vi "open-class-private-data-edit-time.vi"(6 "Mouse Position":T1, 7 "User VI Ref":refnum<vi>, 8 "Is Multi-select?":bool, 9 "Remaining Items":refnum<vi>[](array[refnum]), 10 "Affected Items":T8, 11 "Menu Refnum":refnum<k9>) -> (3 "Menu Items To Add":T2[](array[typedef]))   [LabVIEW 2022 SP3]
doc: "This VI is part of a plug-in for modifying the LabVIEW shortcut menus. This is the builder VI which is called when the shortcut menu is built. It tells LabVIEW which shortcut menu items to add to the menu."
uses:
  <resource>/plugins/PopupMenus/support/Checkmark Status.ctl
  <resource>/plugins/PopupMenus/support/Relative Position.ctl
  <resource>/plugins/PopupMenus/support/Position In Menu.ctl
  <resource>/plugins/PopupMenus/support/Transaction Control.ctl
  <resource>/plugins/PopupMenus/support/Shortcut Menu Item Definition.ctl
  <resource>/plugins/PopupMenus/support/Enabled Menu Item Status.ctl
  open-class-private-data-edit-time.ctl
  <vilib>/Utility/miscctls.llb/LVPositionTypeDef.ctl
panel:
  # "Rules a popup plug-in must follow:\n* This VI's file name must match the file name of the LLB -- only the file extensions should be different.\n* This VI must have debugging disabled or it will be ignored as a plug-in.\n* For all menu items, \"tag suffix + file name of this VI\" must be less than 240 characters.\n* You can disconnect the \"Affected Items\" from the typedef to make the plug-in load faster. The typedef is only there to assist you in keeping this VI and the execution VI using to the same type.\n* All controls on this panel except \"Affected Items\" are locked to prevent accidental edits. Do not change the types or the names of controls other than the elements inside the \"Affected Items\" cluster.\n* See Context Help for more information on the individual controls."
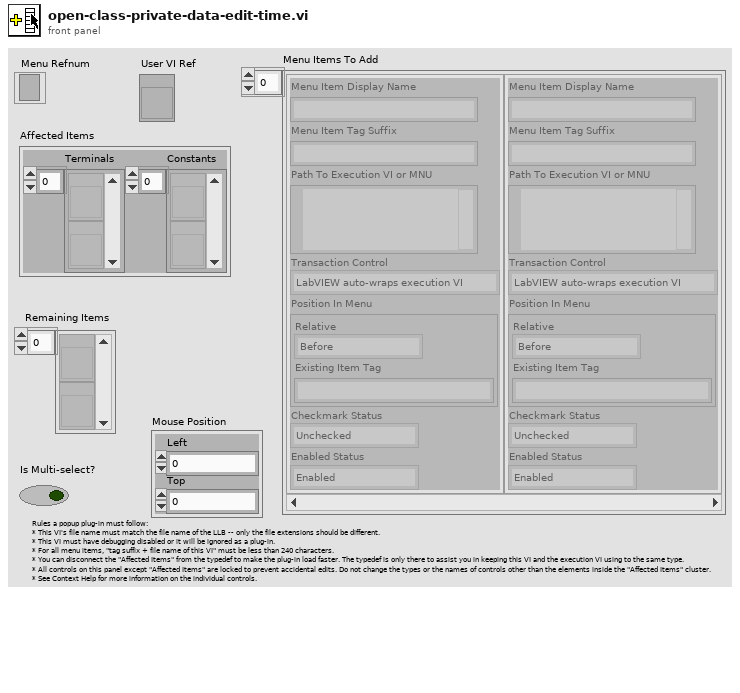
[diagram p1: front panel]
types:
  T1 = typedef "LVPositionTypeDef.ctl" = cluster{"Left":i32, "Top":i32}
  T2 = typedef "Shortcut Menu Item Definition.ctl" = cluster{"Menu Item Display Name":string, "Menu Item Tag Suffix":string, "Path To Execution VI or MNU":path, "Transaction Control":T3, "Position In Menu":T4, "Checkmark Status":T6, "Enabled Status":T7}
  T3 = typedef "Transaction Control.ctl" = enum8{"LabVIEW auto-wraps execution VI", "Execution VI will define if needed"}
  T4 = typedef "Position In Menu.ctl" = cluster{"Relative":T5, "Existing Item Tag":string}
  T5 = typedef "Relative Position.ctl" = enum8{"Before", "Instead of", "After", "Into Submenu"}
  T6 = typedef "Checkmark Status.ctl" = enum8{"Unchecked", "Checked"}
  T7 = typedef "Enabled Menu Item Status.ctl" = enum8{"Enabled", "Disabled"}
  T8 = typedef "open-class-private-data-edit-time.ctl" = cluster{"Terminals":refnum<vi>[], "Constants":refnum<vi>[]}
  T9 = enum32{"not a typedef", "typedef", "strict typedef", "class private data"}
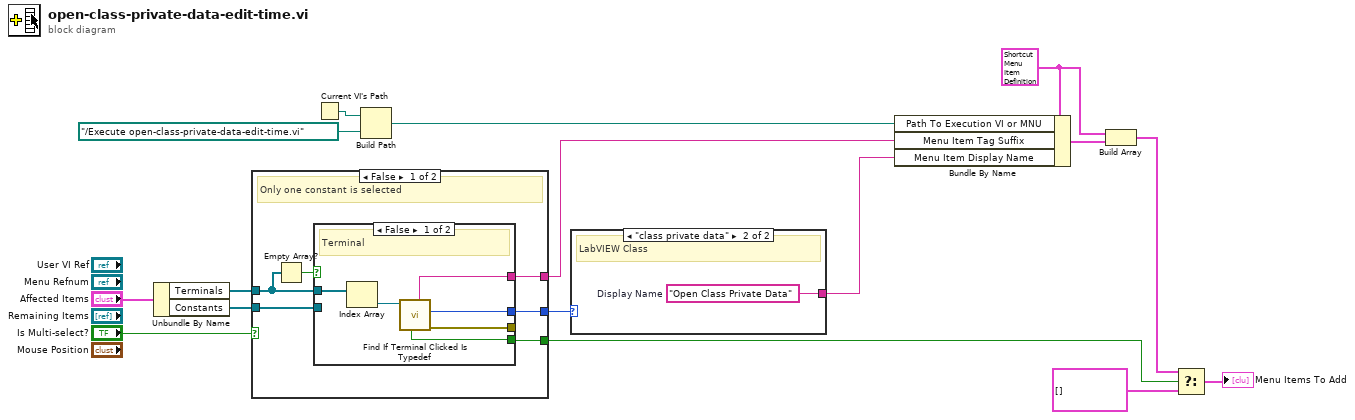
[diagram p0: block diagram]
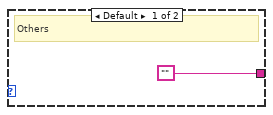
[diagram p2: hidden frame]
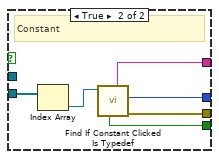
[diagram p3: hidden frame]
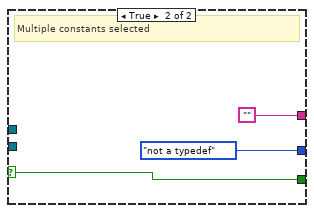
[diagram p4: hidden frame]
diagram:
  w10 = T2 {"Menu Item Display Name"="", "Menu Item Tag Suffix"="", "Path To Execution VI or MNU"=path "", "Transaction Control"=enum."LabVIEW auto-wraps execution VI", "Position In Menu"={"Relative"=enum."Before", "Existing Item Tag"=""}, "Checkmark Status"=enum."Unchecked", "Enabled Status"=enum."Enabled"} ("Cluster")
  n1 = Unbundle By Name("Affected Items") -> ("Terminals"=w12:refnum<vi>[], "Constants"=w11:refnum<vi>[])
  n2 = case shown="False" "Is Multi-select?" {
    selector: "Is Multi-select?" -> [_ w37]
    tunnel: w12 -> [w18 _]
    tunnel: [w22 w37] -> w4
    tunnel: [w21 ""] -> w6
    tunnel: [w20 T9."not a typedef" ("Is Typedef?")] -> w7
    tunnel: w11 -> [w17 _]
    frame False {
      # "Only one constant is selected"
      n3 = Empty Array?(array=w18) -> (empty?=w19:bool)
      n4 = case shown="False" w19 {
        tunnel: [w28 w30] -> w22
        tunnel: [w27 w32] -> w21
        tunnel: [w26 w31] -> w20
        tunnel: w18 -> [w25 _]
        tunnel: w17 -> [_ w33]
        tunnel: [w24 w29] -> _
        frame False {
          # "Terminal"
          n5 = Index Array(array=w25) -> (element=w23:refnum<vi>)  [unwired: 1 in]
          n6 = call "Find If Terminal Clicked Is Typedef.vi"("Terminal In"=w23) -> ("error out"=w24:errorcluster, "Is Typedef?"=w26:T9, "Type Definition/Class Path"=w27:string, "Is Typedef/Class?"=w28:bool)  [unwired: 4 in, 1 out]
        }
        frame True {
          # "Constant"
          n7 = Index Array(array=w33) -> (element=w34:refnum<vi>)  [unwired: 1 in]
          n8 = call "Find If Constant Clicked Is Typedef.vi"("Constant In"=w34) -> ("error out"=w29:errorcluster, "Is Typedef?"=w31:T9, "Type Definition/Class Path"=w32:string, "Is Typedef/Class?"=w30:bool)  [unwired: 4 in, 1 out]
        }
      }
    }
    frame True {
      # "Multiple constants selected"
    }
  }
  n9 = Current VI's Path() -> (path=w13:path)
  n10 = Build Path(base path=w13, name or relative path=path "../Execute open-class-private-data-edit-time.vi" ("execute path")) -> (appended path=w15:path)
  n11 = case shown="\"class private data\"" w7 {
    tunnel: ["" w39] -> w5
    frame Default {
      # "Others"
    }
    frame "class private data" {
      w39 = "Open Class Private Data"  # Display Name
      # "LabVIEW Class"
    }
  }
  n12 = Bundle By Name(cluster=w10, "Path To Execution VI or MNU"=w15, "Menu Item Tag Suffix"=w6, "Menu Item Display Name"=w5) -> (w14:T2)
  n13 = Build Array(w10, w14) -> (w3:T2[])
  n14 = Select(t=w3, s=w4, f=T2[] []) -> (s? t:f=→"Menu Items To Add":T2[])
